vi "Test_GetAndCloseNestedGlobalLogInstance_GlobalLogInstancePersisted.vi"(8 "error in (no error)":errorcluster, 11 "TestCase in":refnum<class "TestComposedLog.lvclass">) -> (0 "error out":errorcluster, 3 "TestCase out":refnum<class "TestComposedLog.lvclass">)   [LabVIEW 2017, in "TestComposedLog.lvclass"]
uses:
  TestComposedLog.lvclass
  Source/Composed Log/Types/Log Level.ctl
  Source/LVQueue Sink/LVQueue Sink.lvclass/LVQueue Sink.ctl
  Source/Composed Log/LoggerReference/LoggerReference.lvclass/LoggerReference.ctl
  26ac907e-b197-4f92-b50b-edca335a3ee8.vi
  26ac907e-b197-4f92-b50b-edca335a3ee8.vi/98f69271-1de1-4081-8ac1-8b840b0807ac.vi
  Source/Composed Log/Singleton Event Log/Get Nested Global Log Instance.vi/b2f05d58-65df-4e80-8f90-78513ac31376.vi
  Source/Composed Log/LoggerReference/Return Aggregate Queues.vi
  Source/Composed Log/LoggerReference/Add Aggregate Log.vi
  26ac907e-b197-4f92-b50b-edca335a3ee8.vi/98f69271-1de1-4081-8ac1-8b840b0807ac.vi/bbd2f978-e444-4445-9202-4eeb40a61ae4.vi
  Source/Composed Log/Singleton Event Log/Get Nested Global Log Instance.vi/b2f05d58-65df-4e80-8f90-78513ac31376.vi/e1ecde32-be62-4caa-aa7a-1c02d969ae2d.vi
  Source/Composed Log/LoggerReference/Log.vi
  Source/Composed Log/LoggerReference/Get Valid Event Time.vi
  Source/Composed Log/LoggerReference/Send Add Sink.vi
  Source/Composed Log/LoggerReference/Remove Stale Logs.vi
  Source/LVQueue Sink/LVQueue Sink.lvclass
  C:/CS/Internal/LabVIEW/Logger/Source/Composed Log/Log Sink/Log Sink.lvclass
  Source/Composed Log/Application Logger/Launch Worker Loop.vi
  Source/Composed Log/LoggerReference/Initialize Logger Instance.vi
  Source/Composed Log/Singleton Event Log/Logger Queue FGV.vi
  Source/Composed Log/Singleton Event Log/Shared Instance FGV.vi
  Source/Composed Log/IErrorFormat/IErrorFormat.lvclass
  Source/Composed Log/LoggerReference/LoggerReference.lvclass
  Source/Composed Log/Log Sink/Log Sink.lvclass
  <vilib>/addons/_JKI Toolkits/VI Tester/TestCase.llb/TestCase.lvclass
  Source/Composed Log/Composed Log.lvlib
  Source/Composed Log/Singleton Event Log/Singleton Event Log.lvlib
  C:/Program Files (x86)/National Instruments/LabVIEW 2017/vi.lib/addons/_JKI Toolkits/VI Tester/TestCase.llb/TestCase.lvclass
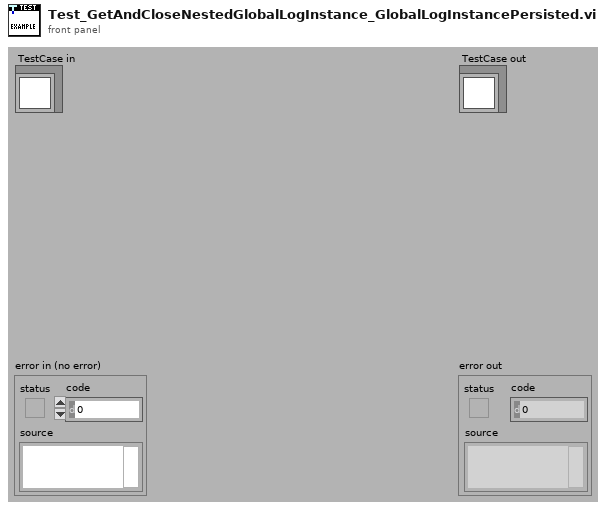
[diagram p1: front panel]
types:
  T1 = typedef "Composed Log.lvlib/Log Level.ctl" = enum16{"Debug", "Info", "Warning", "Error", "Critical"}
  T2 = typedef "Composed Log.lvlib/Log Packet.ctl" = cluster{"Data To Log":string, "Source":string, "Event Level":T1, "Event Time":timestamp}
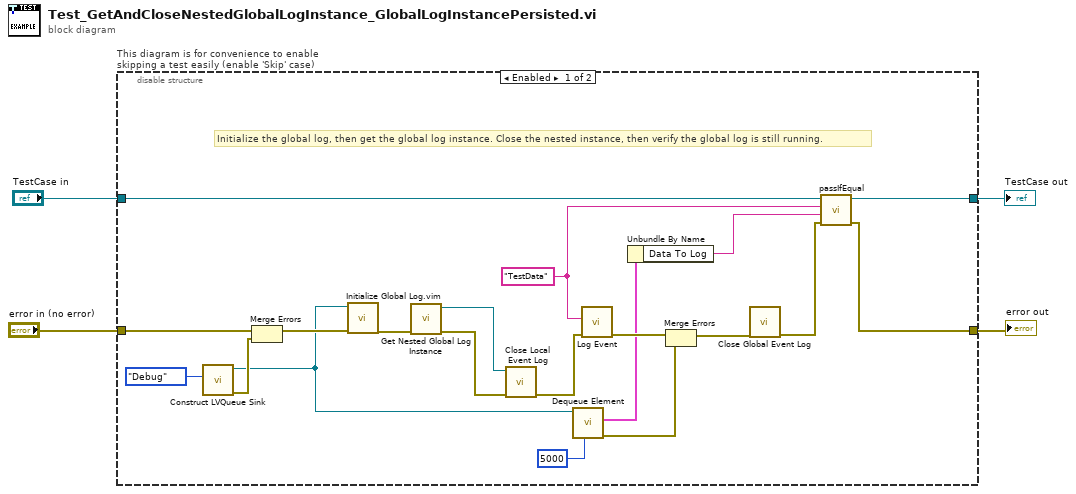
[diagram p0: block diagram]
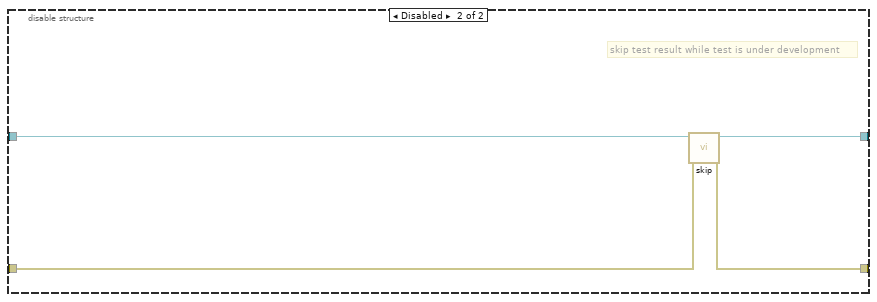
[diagram p2: hidden frame]
diagram:
  n1 = disable-structure "This diagram is for convenience to enable skipping a test easily (enable 'Skip' case)" shown="Enabled" {
    disable-tunnel: "TestCase in" -> [w18 w28]
    disable-tunnel: [w15 w26] -> w1
    disable-tunnel: [w16 w27] -> w3
    disable-tunnel: "error in (no error)" -> [w24 w25]
    frame Enabled {
      w9 = "TestData" ("Data To Log")
      # "Initialize the global log, then get the global log instance. Close the nested instance, then verify the global log is still running."
      n2 = call "Construct LVQueue Sink.vi"("LogLevel"=Log_Level."Debug") -> ("error out"=w22:errorcluster, "LVQueue Sink out"=w10:refnum<class "LVQueue Sink.lvclass">)  [unwired: 9 in]
      n3 = Merge Errors(w24, w22) -> (w21:errorcluster)
      n4 = call "Initialize Global Log.vim"("error in (no error)"=w21, "Log Sink(s)"=w10) -> ("error out"=w20:errorcluster)  [unwired: 8 in, 1 out]
      n5 = call "Get Nested Global Log Instance.vi"("error in (no error)"=w20) -> ("error out"=w19:errorcluster, "Nested Global Log Instance Reference"=w14:refnum<class "LoggerReference.lvclass">)  [unwired: 9 in]
      n6 = call "Close Local Event Log.vi"("error in (no error)"=w19, "Log Instance"=w14) -> ("error out"=w13:errorcluster)  [unwired: 9 in]
      n7 = call "Dequeue Element.vi"("timeout in ms (-1)"=5000, "LVQueue Sink in"=w10) -> ("error out"=w5:errorcluster, "Log Packet"=w8:T2)  [unwired: 6 in, 2 out]
      n8 = call "Log Event.vi"("error in (no error)"=w13, "Data To Log"=w9) -> ("error out"=w12:errorcluster)  [unwired: 9 in]
      n9 = Unbundle By Name(w8) -> ("Data To Log"=w7:string)
      n10 = Merge Errors(w12, w5) -> (w6:errorcluster)
      n11 = call "Close Global Event Log.vi"("error in (no error)"=w6) -> ("error out"=w17:errorcluster)  [unwired: 10 in]
      n12 = call-dynamic "passIfEqual.vi"("error in (no error)"=w17, "y"=w7, "x"=w9, "TestCase in"=w18) -> ("error out"=w16:errorcluster, "TestCase out"=w15:refnum<class "TestComposedLog.lvclass">)  [unwired: 6 in]
    }
    frame Disabled {
      # "skip test result while test is under development"
      n13 = call <vilib>:"skip.vi"("error in (no error)"=w25, "TestCase in"=w28) -> ("error out"=w27:errorcluster, "TestCase out"=w26:refnum<class "TestComposedLog.lvclass">)  [unwired: 8 in]
    }
  }
  "error out" <- w3
  "TestCase out" <- w1
